vi "SingleShot.vi"(8 "error in (no error)":errorcluster, 11 "CameraTesting in":refnum<class "CameraTesting.lvclass">) -> (0 "error out":errorcluster, 3 "CameraTesting out":refnum<class "CameraTesting.lvclass">)   [LabVIEW 2020, in "CameraTesting.lvlib" / "CameraTesting.lvclass"]
uses:
  CameraTesting.lvclass
  CameraTesting.lvclass/CameraTesting.ctl
  Camera/ICamera/ICamera/ICamera.lvclass
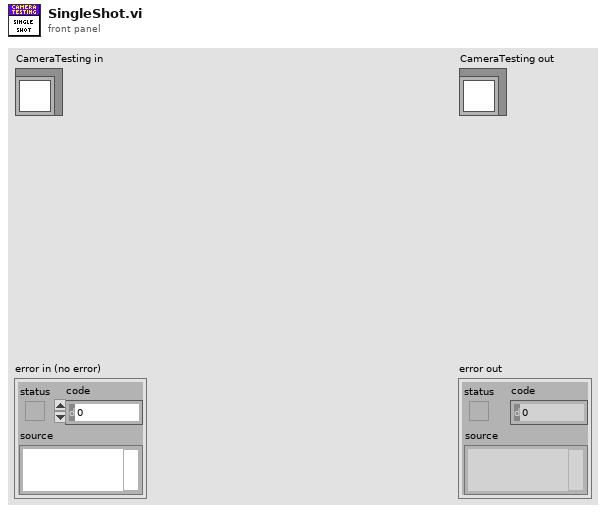
[diagram p1: front panel]
types:
  T1 = typedef "ICamera.lvlib/ICamera.lvclass/SnapInfo.ctl" = cluster{"image depth":i32, "PixelData":u8[], "Bounds":cluster{"Height":i16, "Width":i16}}
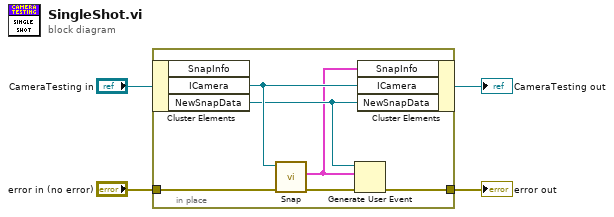
[diagram p0: block diagram]
diagram:
  n1 = in-place {
    in-place-border: "error in (no error)" -> [w10]
    in-place-border: [w8] -> w1
    n2 = in-place-cluster #1("CameraTesting in") -> ("ICamera"=w7:refnum<class "ICamera.lvclass">, "NewSnapData"=w6:refnum<user-event>)  [unwired: 1 out]
    n3 = call-dynamic "Snap.vi"("error in (no error)"=w10, "ICamera in"=w7) -> ("error out"=w9:errorcluster, "SnapInfo"=w5:T1)  [unwired: 7 in, 1 out]
    n4 = Generate User Event(user event=w6, event data cluster=w5, error in=w9) -> (error out=w8:errorcluster)  [unwired: 1 in, 1 out]
    n5 = in-place-cluster #1("SnapInfo"=w5, "ICamera"=w7, "NewSnapData"=w6) -> (→"CameraTesting out":refnum<class "CameraTesting.lvclass">)
  }
  "error out" <- w1
